vi "Tree Add Item.vi"(8 "error in (no error)":errorcluster, 10 "Item Map":T1, 11 "[V]System Tree View in":refnum<class "[V]System Tree View.lvclass">) -> (0 "error out":errorcluster, 3 "[V]System Tree View out":refnum<class "[V]System Tree View.lvclass">)   [LabVIEW 2020, in "[V]System Tree View.lvlib" / "[V]System Tree View.lvclass"]
uses:
  [V]System Tree View.lvclass
  Control/Tree Item.ctl
  [V]System Tree View.lvclass/[V]System Tree View.ctl
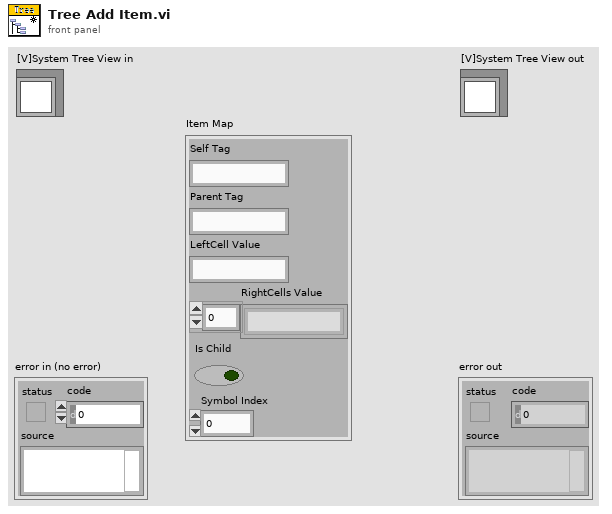
[diagram p1: front panel]
types:
  T1 = typedef "[V]System Tree View.lvlib/[V]System Tree View.lvclass/Tree Item.ctl" = cluster{"Self Tag":string, "Parent Tag":string, "LeftCell Value":string, "RightCells Value":string[], "Is Child":bool, "Symbol Index":i32}
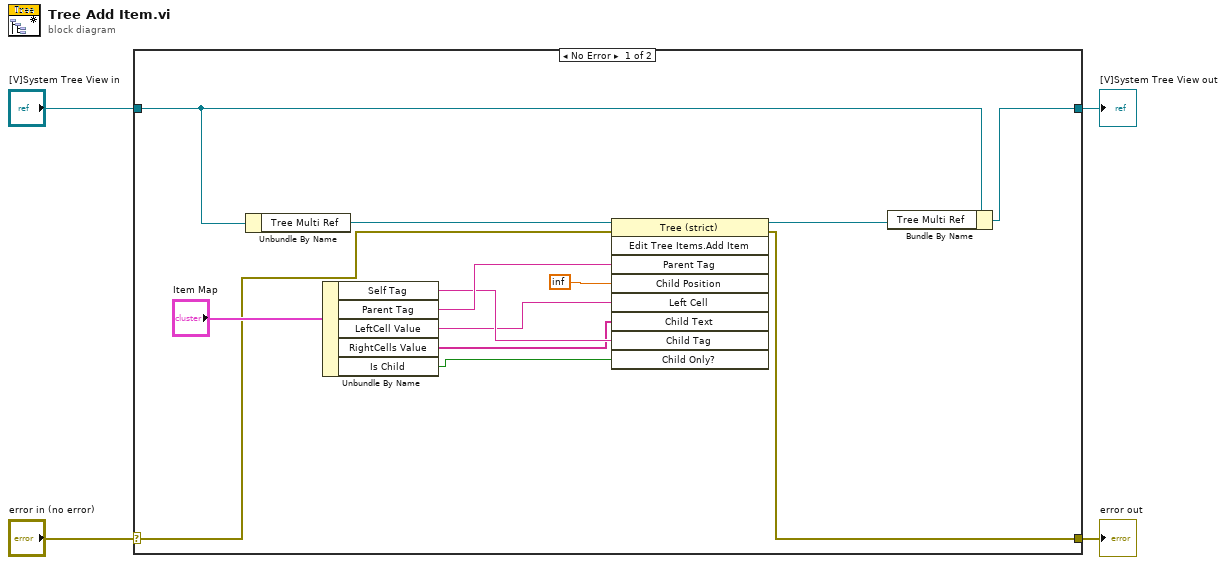
[diagram p0: block diagram]
diagram:
  n1 = case shown="No Error" "error in (no error)" {
    selector: "error in (no error)" -> [w6 w19]
    tunnel: [w5 w19] -> w3
    tunnel: [w15 w18] -> w1
    tunnel: "[V]System Tree View in" -> [w17 w18]
    frame No Error {
      n2 = Unbundle By Name(w17) -> ("Tree Multi Ref"=w14:refnum<vi>)
      n3 = Unbundle By Name("Item Map") -> ("Self Tag"=w10:string, "Parent Tag"=w11:string, "LeftCell Value"=w9:string, "RightCells Value"=w8:string[], "Is Child"=w7:bool)
      n4 = invoke class="Tree (strict)" method="Edit Tree Items.Add Item"(reference=w14, error in=w6, "Parent Tag"=w11, "Child Position"=inf, "Left Cell"=w9, "Child Text"=w8, "Child Tag"=w10, "Child Only?"=w7) -> (reference out=w16:refnum<vi>, error out=w5:errorcluster)  [unwired: 1 in, 7 out]
      n5 = Bundle By Name(cluster=w17, "Tree Multi Ref"=w16) -> (w15:refnum<class "[V]System Tree View.lvclass">)
    }
    frame Error {
    }
  }
  "error out" <- w3
  "[V]System Tree View out" <- w1
